vi "Configure.vi"(8 "error in (no error)":errorcluster, 11 "MeritFactor in":refnum<class "MeritFactor.lvclass">) -> (0 "error out":errorcluster, 2 "cancelled?":bool, 3 "MeritFactor out":refnum<class "MeritFactor.lvclass">)   [LabVIEW 2012, in "MeritFactor.lvclass"]
doc: "The configure method configures the details for the RabbitMQ connection. \n\nIn the derived class, make a call to the parent for setting these parameters."
uses:
  MeritFactor.lvclass
  merit factor type.ctl
  <vilib>/Utility/miscctls.llb/LVPointTypeDef.ctl
  MeritFactor.lvclass/MeritFactor.ctl
  <vilib>/Distrio/Murmex/Murmex/Murmex.lvclass
panel:
  in  "button::configure murmex":bool
  in  "button::cancel":bool
  in  "button::ok":bool
  in  "Tab Control":enum32{"Merit factor", "Debug"}(tab)
  in  "Merit factor type":T1
  # "RabbitMQ parameters"
  # "Window position"
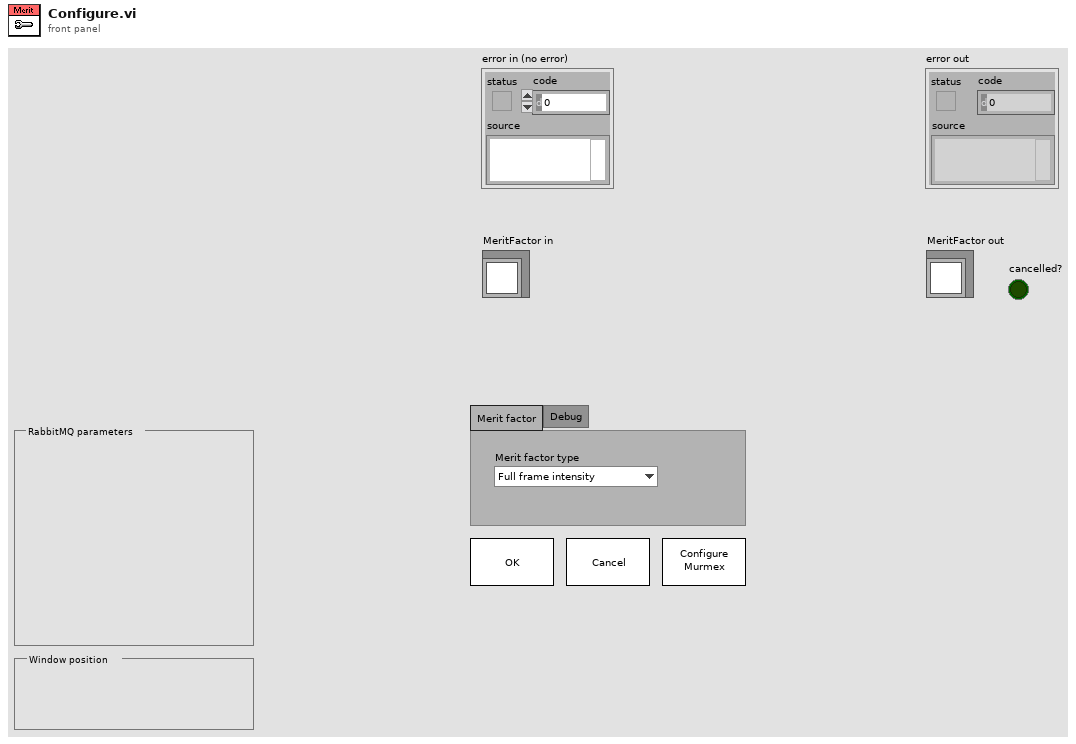
[diagram p1: front panel]
types:
  T1 = typedef "MeritFactor.lvclass/merit factor type.ctl" = enum16{"Full frame intensity", "Brightest pixels intensity", "Contrast (Keller & Stelzer)", "Contrast", "Above-threshold average"}
  T2 = typedef "LVPointTypeDef.ctl" = cluster{"Horizontal":i16, "Vertical":i16}
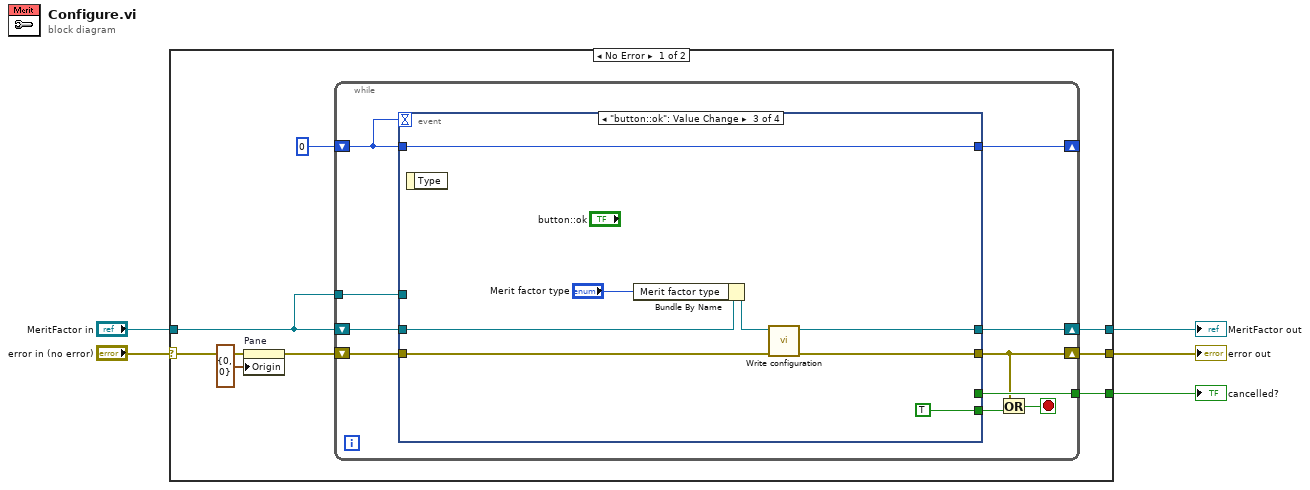
[diagram p0: block diagram]
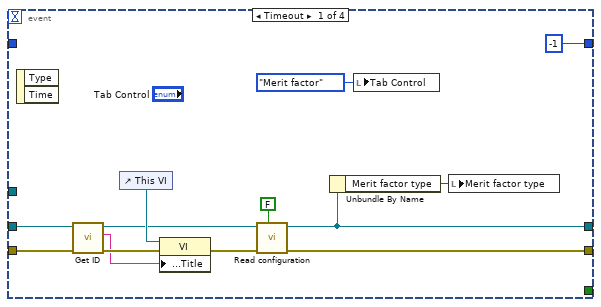
[diagram p2: hidden frame]
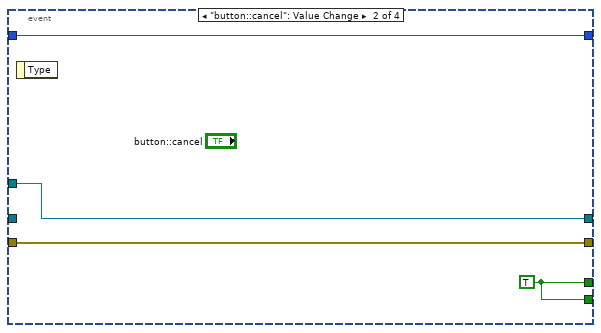
[diagram p3: hidden frame]
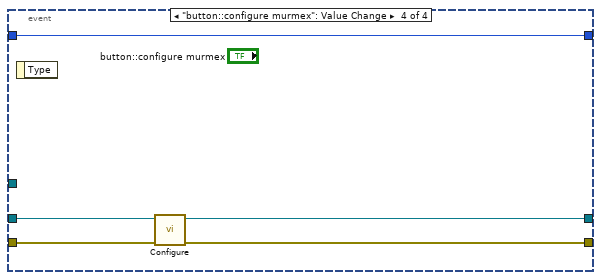
[diagram p4: hidden frame]
diagram:
  n1 = case shown="No Error" "error in (no error)" {
    selector: "error in (no error)" -> [w13 w54]
    tunnel: "MeritFactor in" -> [w9 w55]
    tunnel: [w8 w54] -> w3
    tunnel: [w7 w55] -> w2
    tunnel: [w6 _] -> w1
    frame No Error {
      n2 = property on="Pane" class="Pane"(error in=w13, "Origin"=T2 {"Horizontal"=0, "Vertical"=0}) -> (error out=w11:errorcluster)  [unwired: 1 in, 1 out]
      n3 = while {
        shift-right: [w15] -> w8
        shift-left: w11 -> [w23]
        shift-right: [w21] -> w7
        shift-left: w9 -> [w22]
        shift-right: [w19] -> _
        shift-left: 0 -> [w20]
        tunnel: w9 -> [w18]
        tunnel: [w17] -> w6
        stop <- w14 stop-if-true
        n4 = event shown="[2] \"button::ok\": Value Change" {
          selector: _ -> [_ _ _ _]
          dyn-events: _ -> [_ _ _ _]
          timeout: w20 -> [_ _ _ _]
          tunnel: w23 -> [w36 w39 w48 w53]
          tunnel: w22 -> [w35 _ w45 w52]
          tunnel: [w26 w38 w46 w50] -> w21
          tunnel: w20 -> [_ w40 w43 w49]
          tunnel: [-1 w40 w43 w49] -> w19
          tunnel: w18 -> [_ w38 _ _]
          tunnel: [w25 w39 w47 w51] -> w15
          tunnel: [_ w37 TRUE _] -> w16
          tunnel: [_ w37 _ _] -> w17
          event Timeout {
            n5 = event-data() -> ()  [unwired: 1 in, 2 out]
            n6 = call <vilib>:"Get ID.vi"("error in (no error)"=w36, "Murmex in"=w35) -> ("error out"=w34:errorcluster, "component id"=w32:string, "Murmex out"=w27:refnum<class "MeritFactor.lvclass">)  [unwired: 7 in]
            n7 = control-ref of="This VI"() -> (w33:refnum<vi>)
            n8 = property class="VI"(reference=w33, error in=w34, "Front Panel.Title"=w32) -> (error out=w28:errorcluster)  [unwired: 1 out]
            n9 = call-dynamic "Read configuration.vi"("force loading?"=FALSE, "error in (no error)"=w28, "MeritFactor in"=w27) -> ("error out"=w25:errorcluster, "MeritFactor out"=w26:refnum<class "MeritFactor.lvclass">)  [unwired: 7 in]
            n10 = Unbundle By Name(w26) -> ("Merit factor type"=w31:T1)
            n11 = local write "Tab Control"(enum32{"Merit factor", "Debug"}."Merit factor" ("Tab Control")) -> ()
            n12 = local write "Merit factor type"(w31) -> ()
          }
          event "button::cancel": Value Change {
            w37 = TRUE
            n13 = event-data() -> ()  [unwired: 1 in, 1 out]
          }
          event "button::ok": Value Change {
            n14 = event-data() -> ()  [unwired: 1 in, 1 out]
            n15 = Bundle By Name(cluster=w45, "Merit factor type"="Merit factor type") -> (w44:refnum<class "MeritFactor.lvclass">)
            n16 = call-dynamic "Write configuration.vi"("error in (no error)"=w48, "MeritFactor in"=w44) -> ("error out"=w47:errorcluster, "MeritFactor out"=w46:refnum<class "MeritFactor.lvclass">)  [unwired: 8 in]
          }
          event "button::configure murmex": Value Change {
            n17 = event-data() -> ()  [unwired: 1 in, 1 out]
            n18 = call-parent "Configure.vi"("error in (no error)"=w53, "Murmex in"=w52) -> ("error out"=w51:errorcluster, "Murmex out"=w50:refnum<class "MeritFactor.lvclass">)  [unwired: 7 in, 1 out]
          }
        }
        n19 = Or(x=w15, y=w16) -> (x .or. y?=w14:bool)
      }
    }
    frame Error {
    }
  }
  "error out" <- w3
  "MeritFactor out" <- w2
  "cancelled?" <- w1
